vi "Update Measurement Details [Adv UI].vi"(8 "error in":errorcluster, 9 "measurement service description":string, 10 "measurement service name":string, 11 "project ref":refnum<vi>) -> (0 "error out":errorcluster)   [LabVIEW 2020]
uses:
  MeasurementService Editor.lvlib
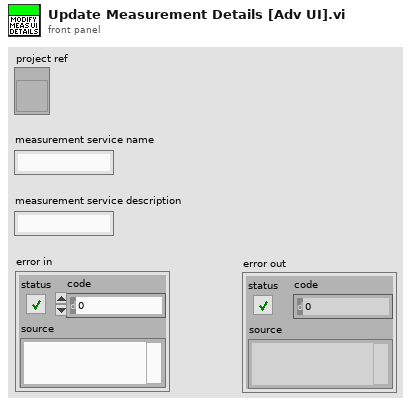
[diagram p1: front panel]
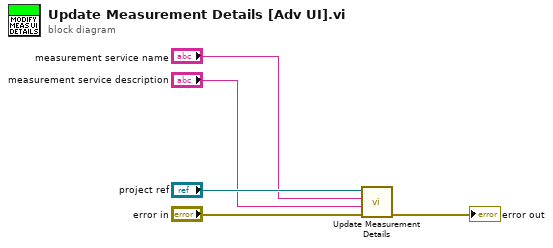
[diagram p0: block diagram]
diagram:
  n1 = call "Update Measurement Details.vi"("error in"="error in", "measurement service description"="measurement service description", "measurement service name"="measurement service name", "project ref"="project ref") -> ("error out"=→"error out":errorcluster)  [unwired: 7 in]
